vi "05_state_machine.vi"() -> ()   [LabVIEW 2017]
uses:
  states_typedef.ctl
panel:
  in  "stop":bool
  in  "Basic Test":bool
  out "Status":string
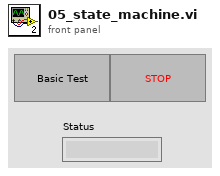
[diagram p1: front panel]
types:
  T1 = typedef "states_typedef.ctl" = enum16{"Init", "Idle", "Basic Test", "Advanced Test", "Notify"}
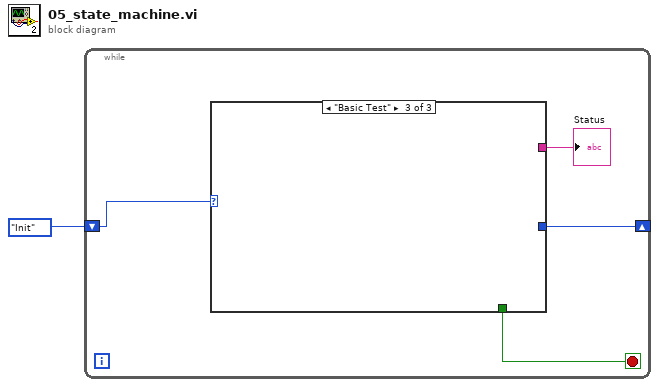
[diagram p0: block diagram]
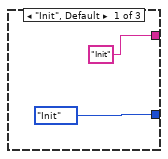
[diagram p2: hidden frame]
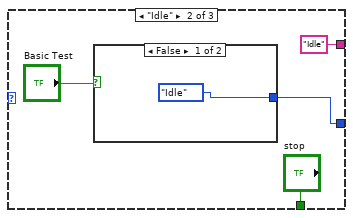
[diagram p3: hidden frame]
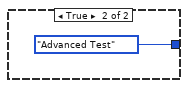
[diagram p4: hidden frame]
diagram:
  n1 = while {
    shift-right: [w4] -> _
    shift-left: states_typedef."Init" -> [w5]
    stop <- w2 stop-if-true
    n2 = case shown="\"Basic Test\"" w5 {
      tunnel: [states_typedef."Init" w9 _] -> w4
      tunnel: ["Init" "Idle" _] -> w3
      tunnel: [_ "stop" _] -> w2
      frame "Init", Default {
      }
      frame "Idle" {
        n3 = case shown="False" "Basic Test" {
          tunnel: [states_typedef."Idle" states_typedef."Advanced Test"] -> w9
          frame False {
          }
          frame True {
          }
        }
      }
      frame "Basic Test" {
      }
    }
    "Status" <- w3
  }
